vi "Receive Control Key Down Event.vi"(8 "error in (no error)":errorcluster, 10 "ControlKeyDownMsg":refnum<class "ControlKeyDownMsg.lvclass">, 11 "IEventAggregator In":refnum<class "IEventAggregator.lvclass">) -> (0 "error out":errorcluster, 3 "IEventAggregator Out":refnum<class "IEventAggregator.lvclass">)   [LabVIEW 2020, in "ActorEvents.lvlib" / "IEventAggregator.lvclass"]
doc: "抽象方法\n接收控件键按下事件"
uses:
  IEventAggregator.lvclass
  IEventAggregator Messages/ControlKeyDownMsg/ControlKeyDownMsg.lvclass
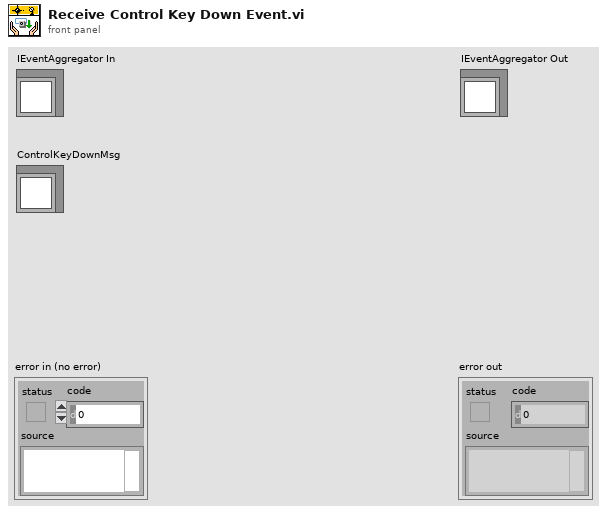
[diagram p1: front panel]
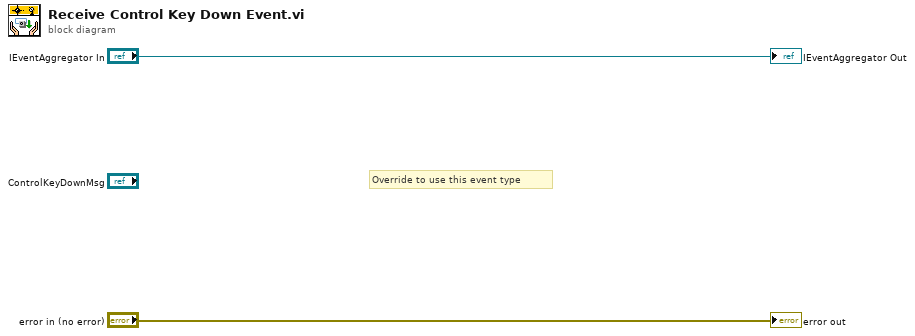
[diagram p0: block diagram]
diagram:
  # "Override to use this event type"
  "error out" <- "error in (no error)"
  "IEventAggregator Out" <- "IEventAggregator In"
